vi "R1SBRControl.vi"(8 "error constant":errorcluster, 11 "LabVIEW Web Service":refnum<class "Web Service.lvclass">) -> (0 "error out":errorcluster)   [LabVIEW 2016]
uses:
  <vilib>/wsapi/Web Service.lvclass
  Controls/R1SBR_SetParams.ctl
  <vilib>/Platform/TimedLoop/XDataNode/timing_clust.ctl
  <vilib>/Platform/TimedLoop/XDataNode/nitl_modes.ctl
  <vilib>/Platform/TimedLoop/XDataNode/wakeup.ctl
  <vilib>/Platform/TimedLoop/XDataNode/loadnilvce.vi
  <vilib>/Platform/TimedLoop/XDataNode/XDataNode.xnode
  <vilib>/Utility/Variable/NI_VariableUtilities.lvlib
  <vilib>/Platform/TimedLoop/XDataNode/XDNodeRunTimeDep.lvlib
panel:
  out "Numeric 2":i32
  out "current time":timestamp
  out "No phases":i32
  out "Numeric":i32
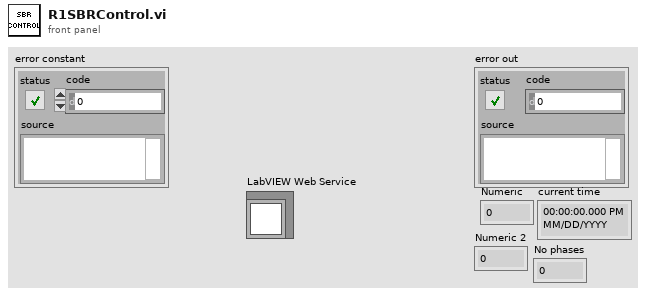
[diagram p1: front panel]
types:
  T1 = typedef "XDNodeRunTimeDep.lvlib/timing_clust.ctl" = cluster{"Expected End [f-1]":u64, "Actual End [f-1]":u64, "Finished Late? [f-1]":bool, "Expected End [i-1]":u64, "Actual End [i-1]":u64, "Finished Late? [i-1]":bool, "Expected Start [i]":u64, "Actual Start [i]":u64, "Expected Start [f]":u64, "Actual Start [f]":u64, "Source Name":string, "Structure Name":string, "Period":i64, "Deadline":i64, "Offset":i64, "Start":i64, "Priority":i32, "Timeout":i32, "Mode":T2, "Wakeup Reason":T3, "Error":errorcluster, "Source Type":string, "Secondary Source Type":string, "Global End Time":u64, "Global Start Time":u64, "Frame Duration":u64, "Iteration Duration":u64, "Assigned CPU":i32, "I/O Scan Engine Mode":u32}
  T2 = typedef "XDNodeRunTimeDep.lvlib/nitl_modes.ctl" = enum32{"No Change", "Process missed periods, maintain original phase", "Discard missed periods, maintain original phase", "Process missed periods, ignore original phase", "Discard missed periods, ignore original phase"}
  T3 = typedef "XDNodeRunTimeDep.lvlib/wakeup.ctl" = enum32{"Normal", "Aborted", "Asynchronous wakeup", "Timing source error", "Timed loop error", "Timeout"}
  T4 = cluster{"Media Pump":bool, "Water Pump":bool, "Effluent Pump":bool, "Release Valve":bool, "Gas Pump":bool}
  T5 = typedef "R1SBR_SetParams.ctl" = cluster{"Phase":string, "Time, min":dbl, "SBR_Manual":cluster{"Media Pump":bool, "Water Pump":bool, "Effluent Pump":bool, "Release Valve":bool, "Gas Pump":bool}}[]
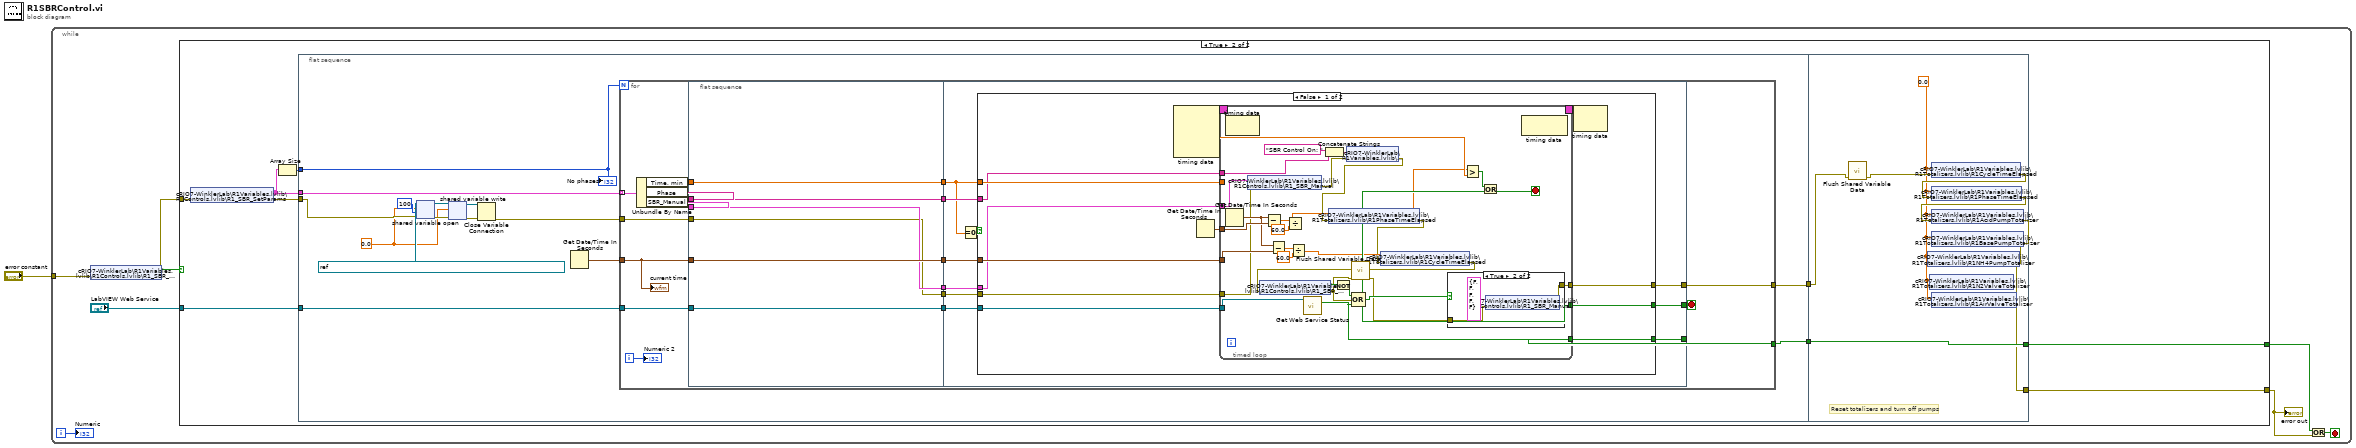
[diagram p0: block diagram]
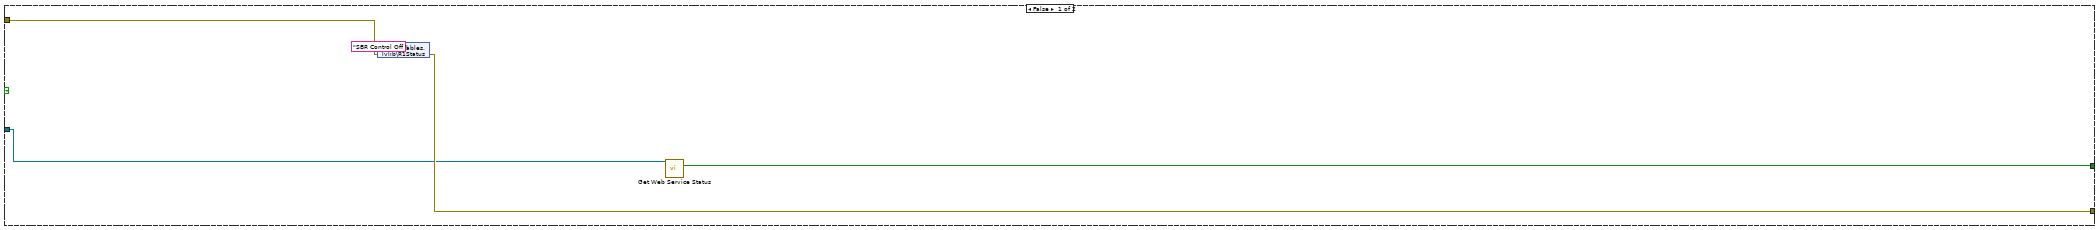
[diagram p2: hidden frame]
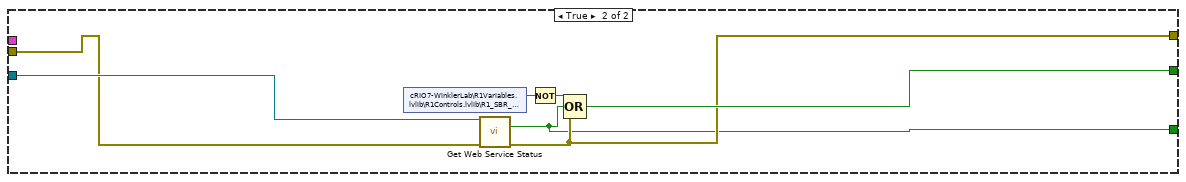
[diagram p4: hidden frame]
diagram:
  n1 = while {
    tunnel: "error constant" -> [w8]
    i -> [w3]
    stop <- w4 stop-if-true
    n2 = shared-variable "cRIO7-WinklerLab\\R1Variables.lvlib\\R1Controls.lvlib\\R1_SBR_Switch"(error in=w8) -> (w9:bool, error out=w7:errorcluster)
    n3 = case shown="True" w9 {
      tunnel: "LabVIEW Web Service" -> [w11 w21]
      tunnel: w7 -> [w13 w20]
      tunnel: [w12 w15] -> w5
      tunnel: [w10 w17] -> w2
      frame False {
        n4 = shared-variable ".\\R1Variables.lvlib\\R1Status"("SBR Control Off " ("string"), error in=w13) -> (error out=w12:errorcluster)
        n5 = call <vilib>:"Get Web Service Status.vi"("LabVIEW Web Service"=w11) -> ("service stopping?"=w10:bool)  [unwired: 12 in, 2 out]
      }
      frame True {
        n6 = shared-variable "cRIO7-WinklerLab\\R1Variables.lvlib\\R1Controls.lvlib\\R1_SBR_SetParams"(error in=w20) -> (w22:T5, error out=w19:errorcluster)
        n7 = Array Size(array=w22) -> (size(s)=w23:i32)
        n8 = flat-sequence {
          tunnel: w22 -> [w37]
          tunnel: w23 -> [w38]
          tunnel: w21 -> [w36]
          tunnel: w19 -> [w27]
          tunnel: [w34] -> w18
          tunnel: [w24] -> w16
          tunnel: w18 -> [w134]
          tunnel: [w132] -> w17
          tunnel: w16 -> [w132]
          tunnel: [w131] -> w15
          frame #0 {
            w25 = 0.0 ("R1CycleTimeElapsed")
            n9 = shared-variable-open(refnum<k21> "ni.var.psp://crio1-winklerlab/R1Variables/R1Totalizers/R1CycleTimeElapsed" ("shared variable refnum in"), w27, w25, 100 ("timeout ms")) -> (w32:refnum<k21>, w30:errorcluster)  [unwired: 2 in]
            n10 = shared-variable-write(w32, w30, w25) -> (w31:refnum<k21>, w29:errorcluster)
            n11 = Close Variable Connection(8:w29, 11:w31) -> (0:w26:errorcluster)
            n12 = Get Date/Time In Seconds() -> (seconds since 1Jan1904=w35:timestamp)
            n13 = for {
              N: w38 -> [_]
              tunnel: w37 -> [w55] mode=indexing
              tunnel: w36 -> [w53]
              tunnel: w26 -> [w47]
              tunnel: [w45] -> w34
              tunnel: w35 -> [w42]
              tunnel: [w41] -> w24
              i -> [w43]
              stop <- w44 stop-if-true
              n14 = Unbundle By Name(w55) -> ("Time, min"=w50:dbl, "Phase"=w49:string, "SBR_Manual"=w54:T4)
              n15 = flat-sequence {
                tunnel: w50 -> [w60]
                tunnel: w54 -> [w57]
                tunnel: w53 -> [w61]
                tunnel: [w61] -> w52
                tunnel: [w60] -> w51
                tunnel: w49 -> [w59]
                tunnel: [w59] -> w48
                tunnel: w47 -> [w56]
                tunnel: w42 -> [w58]
                tunnel: [w58] -> w46
                tunnel: [w57] -> w40
                tunnel: [w56] -> w39
                tunnel: [w70] -> w44
                tunnel: w52 -> [w71]
                tunnel: w51 -> [w62]
                tunnel: w48 -> [w69]
                tunnel: w46 -> [w68]
                tunnel: [w67] -> w45
                tunnel: [w66] -> w41
                tunnel: w40 -> [w65]
                tunnel: w39 -> [w64]
                frame #0 {
                }
                frame #1 {
                  n16 = Equal To 0?(x=w62) -> (x = 0?=w63:bool)
                  n17 = case shown="False" w63 {
                    tunnel: w71 -> [w83 w125]
                    tunnel: [w82 w123] -> w70
                    tunnel: w69 -> [w72 _]
                    tunnel: w68 -> [w80 _]
                    tunnel: [w79 w122] -> w67
                    tunnel: [w78 w121] -> w66
                    tunnel: w65 -> [w73 _]
                    tunnel: w64 -> [w74 w124]
                    tunnel: w62 -> [w77 _]
                    frame False {
                      n18 = node-c288() -> (w76:T1)  [unwired: 4 in]
                      n19 = Get Date/Time In Seconds() -> (seconds since 1Jan1904=w81:timestamp)
                      n20 = timed-loop {
                        tunnel: w83 -> [w105]
                        tunnel: [w100] -> w82
                        tunnel: w81 -> [w109]
                        tunnel: w80 -> [w106]
                        tunnel: [w98] -> w79
                        tunnel: [w101] -> w78
                        tunnel: w74 -> [w87]
                        tunnel: w77 -> [w97]
                        timing: w76 -> [_]
                        timing-out: [_] -> w75
                        tunnel: w73 -> [w85]
                        tunnel: w72 -> [w84]
                        stop <- w96 stop-if-true
                        n21 = node-c288() -> ()  [unwired: 1 in, 1 out]
                        n22 = Get Date/Time In Seconds() -> (seconds since 1Jan1904=w107:timestamp)
                        n23 = shared-variable "cRIO7-WinklerLab\\R1Variables.lvlib\\R1Controls.lvlib\\R1_SBR_Manual"(w85, error in=w87) -> (error out=w88:errorcluster)
                        n24 = Subtract(x=w107, y=w109) -> (x-y=w110:dbl)
                        n25 = Subtract(x=w107, y=w106) -> (x-y=w104:dbl)
                        n26 = Divide(x=w110, y=60.0) -> (x/y=w94:dbl)
                        n27 = Divide(x=w104, y=60.0) -> (x/y=w93:dbl)
                        n28 = call <vilib>:"Get Web Service Status.vi"("LabVIEW Web Service"=w105) -> ("service stopping?"=w101:bool)  [unwired: 12 in, 2 out]
                        n29 = Concatenate Strings("SBR Control On: " ("string"), w84) -> (w89:string)
                        n30 = shared-variable "cRIO7-WinklerLab\\R1Variables.lvlib\\R1Status"(w89, error in=w88) -> (error out=w86:errorcluster)
                        n31 = shared-variable "cRIO7-WinklerLab\\R1Variables.lvlib\\R1Totalizers.lvlib\\R1PhaseTimeElapsed"(w94, error in=w86) -> (error out=w91:errorcluster)
                        n32 = shared-variable "cRIO7-WinklerLab\\R1Variables.lvlib\\R1Totalizers.lvlib\\R1CycleTimeElapsed"(w93, error in=w91) -> (error out=w92:errorcluster)
                        n33 = shared-variable "cRIO7-WinklerLab\\R1Variables.lvlib\\R1Controls.lvlib\\R1_SBR_Switch"(error in=w92) -> (w112:bool, error out=w102:errorcluster)
                        n34 = Not(x=w112) -> (.not. x?=w111:bool)
                        n35 = call <vilib>:"Flush Shared Variable Data.vi"("error in (no error)"=w102) -> ("error out"=w99:errorcluster)  [unwired: 10 in]
                        n36 = Compound Arithmetic op=OR(w111, w102, w101) -> (w100:bool)
                        n37 = case shown="True" w100 {
                          tunnel: w99 -> [w115 w117]
                          tunnel: [w115 w116] -> w98
                          frame False {
                          }
                          frame True {
                            n38 = shared-variable "cRIO7-WinklerLab\\R1Variables.lvlib\\R1Controls.lvlib\\R1_SBR_Manual"(T4 {"Media Pump"=FALSE, "Water Pump"=FALSE, "Effluent Pump"=FALSE, "Release Valve"=FALSE, "Gas Pump"=FALSE} ("R1SBRManual"), error in=w117) -> (error out=w116:errorcluster)
                          }
                        }
                        n39 = Greater?(x=w94, y=w97) -> (0:w95:bool)
                        n40 = Or(x=w95, y=w100) -> (x .or. y?=w96:bool)
                        n41 = node-c288() -> ()  [unwired: 1 in, 1 out]
                      }
                      n42 = node-c288(w75) -> ()  [unwired: 1 out]
                    }
                    frame True {
                      n43 = shared-variable "cRIO7-WinklerLab\\R1Variables.lvlib\\R1Controls.lvlib\\R1_SBR_Switch"() -> (w127:bool)  [unwired: 1 in, 1 out]
                      n44 = call <vilib>:"Get Web Service Status.vi"("LabVIEW Web Service"=w125, "error in (no error)"=w124) -> ("service stopping?"=w121:bool, "error out"=w122:errorcluster)  [unwired: 11 in, 1 out]
                      n45 = Not(x=w127) -> (.not. x?=w126:bool)
                      n46 = Compound Arithmetic op=OR(w126, w121, w122) -> (w123:bool)
                    }
                  }
                }
              }
              "Numeric 2" <- w43
              "current time" <- w42
            }
            "No phases" <- w38
          }
          frame #1 {
            w128 = 0.0 ("R1CycleTimeElapsed")
            # "Reset totalizers and turn off pumps"
            n47 = call <vilib>:"Flush Shared Variable Data.vi"("error in (no error)"=w134) -> ("error out"=w133:errorcluster)  [unwired: 10 in]
            n48 = shared-variable "cRIO7-WinklerLab\\R1Variables.lvlib\\R1Totalizers.lvlib\\R1N2ValveTotalizer"(w128) -> ()  [unwired: 1 in, 1 out]
            n49 = shared-variable "cRIO7-WinklerLab\\R1Variables.lvlib\\R1Totalizers.lvlib\\R1CycleTimeElapsed"(w128, error in=w133) -> (error out=w136:errorcluster)
            n50 = shared-variable "cRIO7-WinklerLab\\R1Variables.lvlib\\R1Totalizers.lvlib\\R1PhaseTimeElapsed"(w128, error in=w136) -> (error out=w135:errorcluster)
            n51 = shared-variable "cRIO7-WinklerLab\\R1Variables.lvlib\\R1Totalizers.lvlib\\R1AcidPumpTotalizer"(w128, error in=w135) -> (error out=w130:errorcluster)
            n52 = shared-variable "cRIO7-WinklerLab\\R1Variables.lvlib\\R1Totalizers.lvlib\\R1BasePumpTotalizer"(w128, error in=w130) -> (error out=w129:errorcluster)
            n53 = shared-variable "cRIO7-WinklerLab\\R1Variables.lvlib\\R1Totalizers.lvlib\\R1NH4PumpTotalizer"(w128, error in=w129) -> (error out=w131:errorcluster)
            n54 = shared-variable "cRIO7-WinklerLab\\R1Variables.lvlib\\R1Totalizers.lvlib\\R1AirValveTotalizer"(w128) -> ()  [unwired: 1 in, 1 out]
          }
        }
      }
    }
    "error out" <- w5
    n55 = Or(x=w2, y=w5) -> (x .or. y?=w4:bool)
    "Numeric" <- w3
  }
